vi "LineToSetting.vi"(8 "Scale":i32[](array[numeric])=[1460000, 1460000, 700], 9 "GridSize":dbl=5.0, 10 "Line":dbl[](array[numeric])=[30.0, 30.0, 50.0, 50.0, 15.0], 11 "Scan Settings":T1={"XStart"=-150000000, "XEnd"=150000000, "XNum"=350, "YStart"=-150000000, "YEnd"=150000000, "YNum"=500, "ZStart"=-30000, "ZEnd"=30000, "ZNum"=30}) -> (3 "Settings":i32[][](array[numeric]))   [LabVIEW 2011]
panel:
  in  "ZGain":dbl=2.0
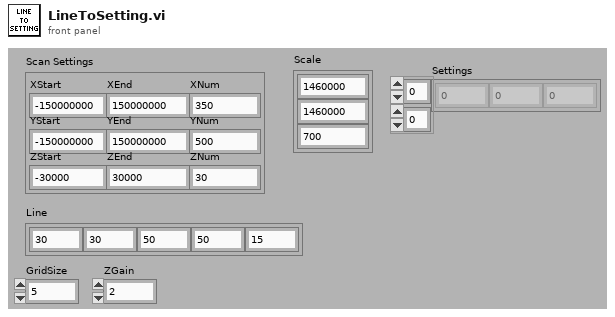
[diagram p1: front panel]
types:
  T1 = cluster{"XStart":i32, "XEnd":i32, "XNum":i32, "YStart":i32, "YEnd":i32, "YNum":i32, "ZStart":i32, "ZEnd":i32, "ZNum":i32}
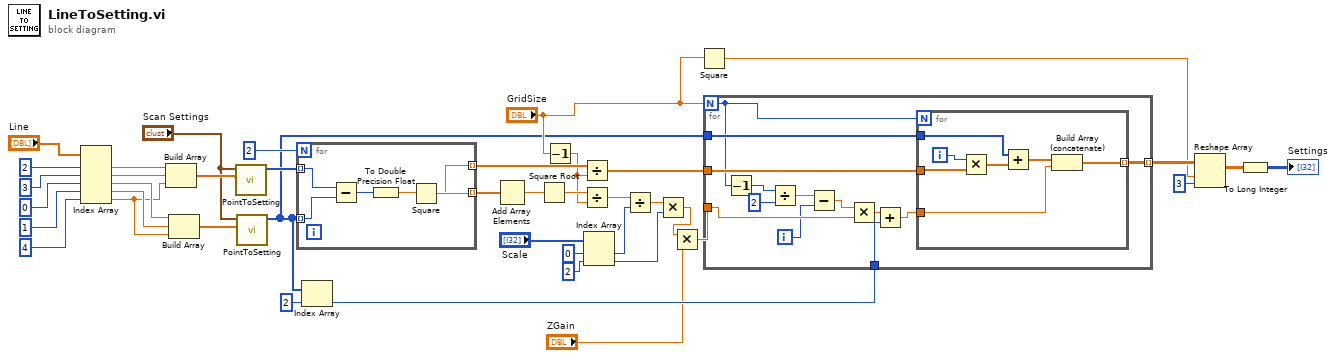
[diagram p0: block diagram]
diagram:
  n1 = Index Array(array="Line", index #1=2 ("index"), index #2=3 ("index"), index #3=0 ("index"), index #4=1 ("index"), index #5=4 ("index")) -> (element #1=w35:dbl, element #2=w34:dbl, element #3=w33:dbl, element #4=w32:dbl, element #5=w31:dbl)
  n2 = Build Array(w35, w34, w31) -> (w9:dbl[])
  n3 = Build Array(w33, w32, w31) -> (w7:dbl[])
  n4 = call "PointToSetting.vi"("Clicked"=w9, "Scan Settings"="Scan Settings") -> ("Setting"=w10:i32[])  [unwired: 9 in]
  n5 = call "PointToSetting.vi"("Clicked"=w7, "Scan Settings"="Scan Settings") -> ("Setting"=w6:i32[])  [unwired: 9 in]
  n6 = for {
    N: 2 -> [_]
    tunnel: w10 -> [w46] mode=indexing
    tunnel: w6 -> [w45] mode=indexing
    tunnel: [w44] -> w30 mode=indexing
    tunnel: [w42] -> w19 mode=indexing
    n7 = Subtract(x=w46, y=w45) -> (x-y=w43:i32)
    n8 = To Double Precision Float(number=w43) -> (double precision float=w42:dbl)
    n9 = Square(x=w42) -> (x^2=w44:dbl)
  }
  n10 = Index Array(array=w6, index=2) -> (element=w4:i32)
  n11 = Add Array Elements(numeric array=w30) -> (sum=w29:dbl)
  n12 = Square Root(x=w29) -> (sqrt(x)=w28:dbl)
  n13 = Decrement(x="GridSize") -> (x-1=w11:dbl)
  n14 = Divide(x=w19, y=w11) -> (x/y=w18:dbl[])
  n15 = Divide(x=w28, y=w11) -> (x/y=w23:dbl)
  n16 = Index Array(array="Scale", index #1=0 ("index"), index #2=2 ("index")) -> (element #1=w22:i32, element #2=w20:i32)
  n17 = Divide(x=w23, y=w22) -> (x/y=w21:dbl)
  n18 = Multiply(x=w21, y=w20) -> (x*y=w3:dbl)
  n19 = Multiply(x=w3, y="ZGain") -> (x*y=w2:dbl)
  n20 = Square(x="GridSize") -> (x^2=w15:dbl)
  n21 = for {
    N: "GridSize" -> [w55]
    tunnel: w2 -> [w56]
    tunnel: w6 -> [w59]
    tunnel: w18 -> [w58]
    tunnel: [w57] -> w17 mode=indexing
    tunnel: w4 -> [w47]
    i -> [w51]
    n22 = Decrement(x=w55) -> (x-1=w54:i32)
    n23 = Divide(x=w54, y=2) -> (x/y=w52:dbl)
    n24 = Subtract(x=w52, y=w51) -> (x-y=w50:dbl)
    n25 = Multiply(x=w50, y=w56) -> (x*y=w49:dbl)
    n26 = Add(x=w49, y=w47) -> (x+y=w48:dbl)
    n27 = for {
      N: w55 -> [_]
      tunnel: w59 -> [w63]
      tunnel: w58 -> [w66]
      tunnel: w48 -> [w61]
      tunnel: [w60] -> w57 mode=indexing
      i -> [w65]
      n28 = Multiply(x=w65, y=w66) -> (x*y=w64:dbl[])
      n29 = Add(x=w63, y=w64) -> (x+y=w62:dbl[])
      n30 = Build Array (concatenate)(w62, w61) -> (w60:dbl[])
    }
  }
  n31 = Reshape Array(w17, w15, 3 ("dimension size")) -> (w14:dbl[][])
  n32 = To Long Integer(number=w14) -> (32bit integer=→"Settings":i32[][])
